vi "Obtain Servicio from paquetes.vi"(8 "error in (no error)":errorcluster, 10 "Servicio seleccionado":string, 11 "Hardware in":refnum<class "Hardware.lvclass">) -> (0 "error out":errorcluster, 3 "Hardware out":refnum<class "Hardware.lvclass">)   [LabVIEW 2020, in "Hardware.lvlib" / "Hardware.lvclass"]
uses:
  Hardware.lvclass
  Hardware.lvclass/Hardware.ctl
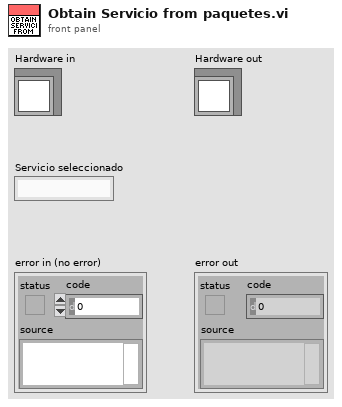
[diagram p1: front panel]
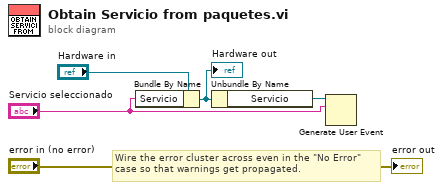
[diagram p0: block diagram]
diagram:
  # "Wire the error cluster across even in the \"No Error\"\ncase so that warnings get propagated."
  n1 = Bundle By Name(cluster="Hardware in", "Servicio"="Servicio seleccionado") -> (w3:refnum<class "Hardware.lvclass">)
  "Hardware out" <- w3
  n2 = Unbundle By Name(w3) -> ("Servicio"=w2:refnum<user-event>)
  n3 = Generate User Event(user event=w2, event data cluster="Servicio seleccionado") -> ()  [unwired: 2 in, 2 out]
  "error out" <- "error in (no error)"
